vi "4155C Filename.vi"() -> ()   [LabVIEW 2019]
panel:
  in  "File info":cluster{"Filename":string, "Directory":path}={"Filename"="", "Directory"=path "D:/Users"}
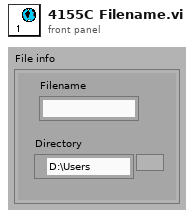
[diagram p1: front panel]
diagram:
